vi "exportFile.vi"(8 "error in":errorcluster, 10 "file path (dialog if empty)":path, 11 "Waveform Graph":waveform(dbl)[](array[waveform])) -> (0 "error out":errorcluster)   [LabVIEW 2013]
uses:
  <vilib>/Analysis/1siggen.llb/Ramp Pattern by Samples.vi
  <vilib>/Utility/file.llb/Write To Spreadsheet File (DBL).vi
  <vilib>/Analysis/NI_AALBase.lvlib
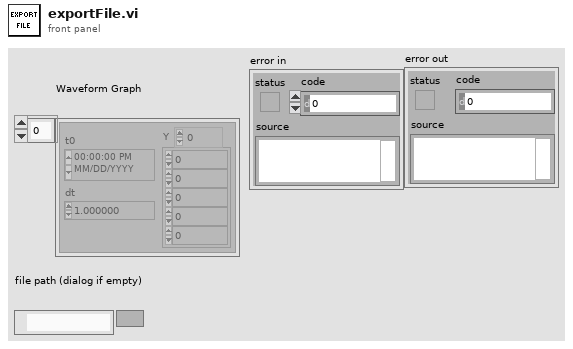
[diagram p1: front panel]
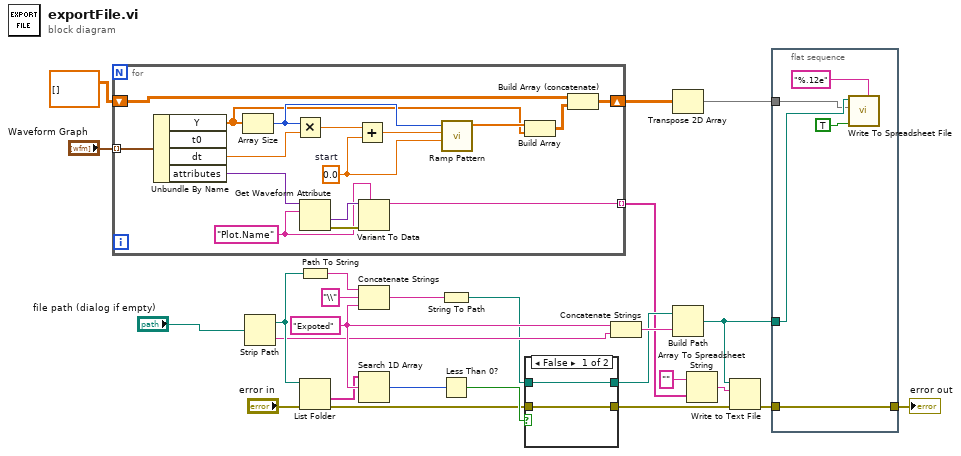
[diagram p0: block diagram]
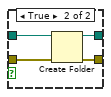
[diagram p2: hidden frame]
diagram:
  w22 = "Expoted"
  n1 = for {
    tunnel: "Waveform Graph" -> [w42] mode=indexing
    shift-right: [w28] -> w6
    shift-left: dbl[][] [] -> [w30]
    tunnel: [w27] -> w8 mode=indexing
    w33 = 0.0  # start
    w38 = "Plot.Name" ("name")
    n2 = Unbundle By Name(w42) -> ("Y"=w31:dbl[], "dt"=w36:dbl, "attributes"=w41:variant)  [unwired: 1 out]
    n3 = Array Size(array=w31) -> (size(s)=w37:i32)
    n4 = Multiply(x=w37, y=w36) -> (x*y=w35:dbl)
    n5 = Get Waveform Attribute(6:w38, 7:w41) -> (0:w40:errorcluster, 1:w39:variant)  [unwired: 2 in, 2 out]
    n6 = Add(x=w35, y=w33) -> (x+y=w34:dbl)
    n7 = Variant To Data(error in=w40, type=w38, Variant=w39) -> (data=w27:string)  [unwired: 1 out]
    n8 = call-poly <vilib>:"Ramp Pattern.vi"("start"=w33, "end"=w34, "samples"=w37) -> ("Ramp Pattern"=w32:dbl[])  [unwired: 7 in, 1 out]
    n9 = Build Array(w32, w31) -> (w29:dbl[][])
    n10 = Build Array (concatenate)(w30, w29) -> (w28:dbl[][])
  }
  n11 = Strip Path(path="file path (dialog if empty)") -> (stripped path=w24:path, name=w21:string)
  n12 = Path To String(path=w24) -> (string=w16:string)
  n13 = List Folder(path=w24, error in="error in") -> (folder names=w12:string[], error out=w3:errorcluster)  [unwired: 2 in, 2 out]
  n14 = Concatenate Strings(w16, "\\" ("string"), w22) -> (w18:string)
  n15 = Search 1D Array(1D array=w12, element=w22) -> (index of element=w13:i32)  [unwired: 1 in]
  n16 = String To Path(string=w18) -> (path=w17:path)
  n17 = Less Than 0?(x=w13) -> (x < 0?=w15:bool)
  n18 = case shown="False" w15 {
    tunnel: w17 -> [w44 w48]
    tunnel: [w44 w47] -> w19
    tunnel: w3 -> [w43 w46]
    tunnel: [w43 w45] -> w2
    frame False {
    }
    frame True {
      n19 = Create Folder(path (use dialog)=w48, error in=w46) -> (created path=w47:path, error out=w45:errorcluster)  [unwired: 1 in, 1 out]
    }
  }
  n20 = Concatenate Strings(w22, w21) -> (w23:string)
  n21 = Transpose 2D Array(2D array=w6) -> (transposed array=w10:dbl[][])
  n22 = Build Path(base path=w19, name or relative path=w23) -> (appended path=w20:path)
  n23 = Array To Spreadsheet String(array=w8, 3:"" ("format string")) -> (spreadsheet string=w11:string)  [unwired: 1 in]
  n24 = Write to Text File(file (use dialog)=w20, text=w11, error in=w2) -> (error out=w9:errorcluster)  [unwired: 1 in, 2 out]
  n25 = flat-sequence {
    tunnel: w20 -> [w53]
    tunnel: w9 -> [w49]
    tunnel: w10 -> [w52]
    tunnel: [w49] -> w1
    frame #0 {
      n26 = call-poly <vilib>:"Write To Spreadsheet File.vi"("format (%.3f)"="%.12e", "append to file? (new file:F)"=TRUE, "2D data"=w52, "file path (dialog if empty)"=w53) -> ()  [unwired: 4 in, 1 out]
    }
  }
  "error out" <- w1
